vi "get_variable.vi"(4 "deviceName":string, 6 "timeout (ms)":i32=10000, 7 "IP address":string, 8 "error in (no error)":errorcluster, 9 "token cluster in":T1, 10 "variable name":string, 11 "client handle":T2) -> (0 "error out":errorcluster, 1 "token cluster":T1, 2 "variable value":string, 3 "client handle out":T2)   [LabVIEW 2018]
uses:
  <vilib>/httpClient/ClientHandle.ctl
  <vilib>/httpClient/LabVIEWHTTPClient.lvlib
panel:
  out "url":string
  out "headers":string
  out "status code":string
  out "msg":string
  out "reponse":string
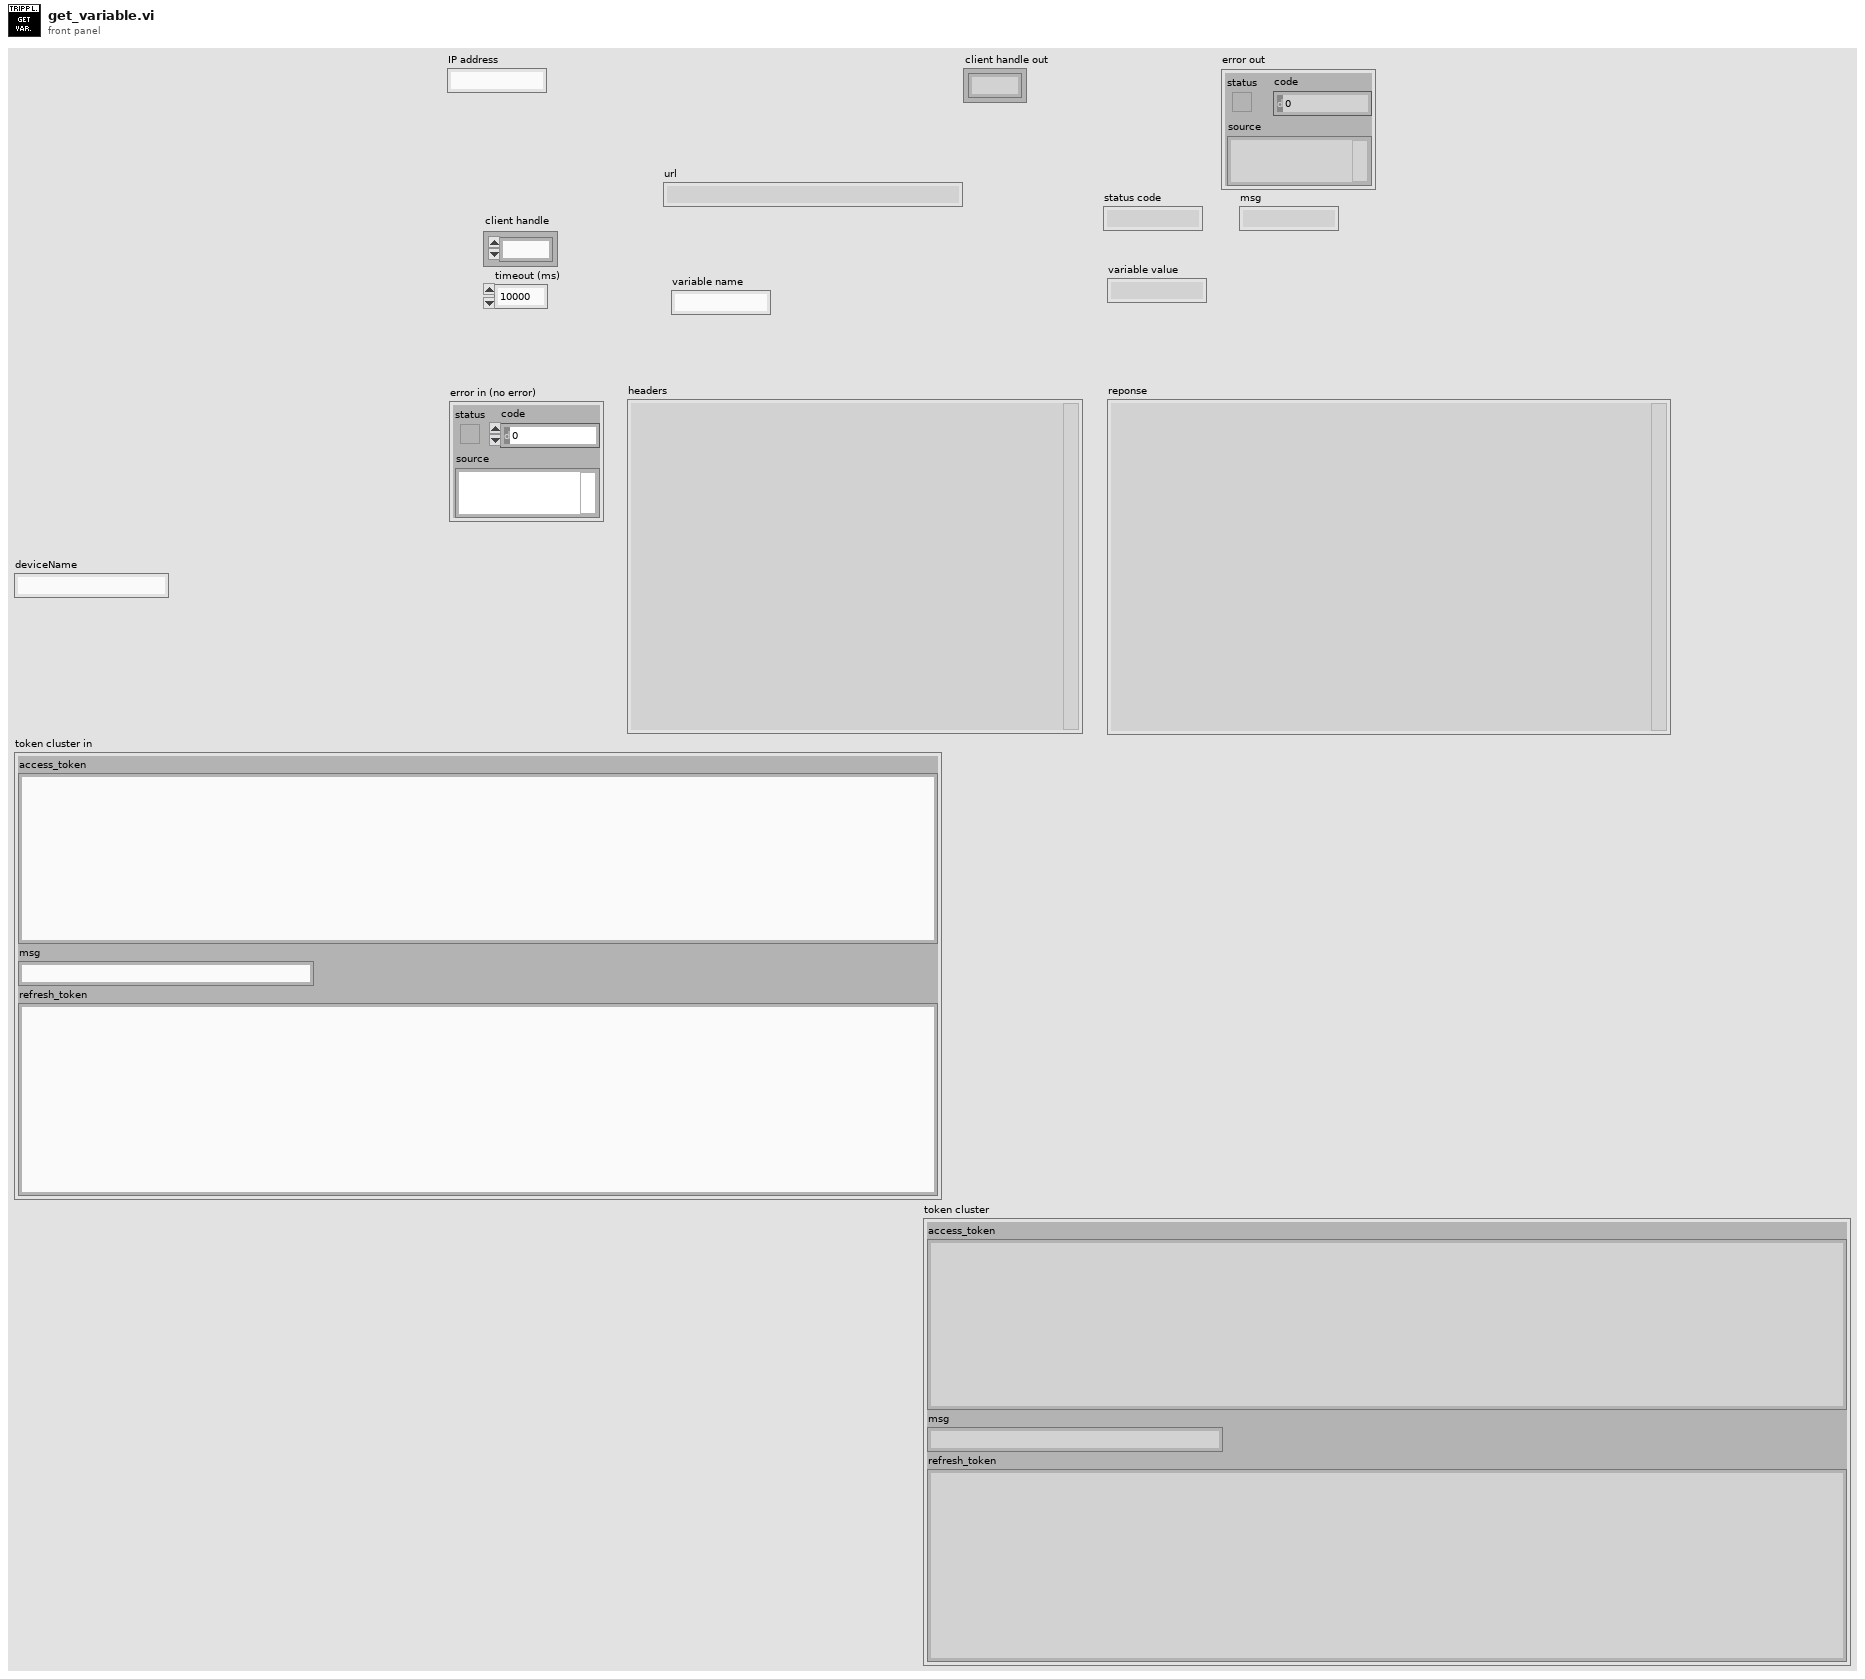
[diagram p1: front panel]
types:
  T1 = cluster{"access_token":string, "msg":string, "refresh_token":string}
  T2 = typedef "LabVIEWHTTPClient.lvlib/ClientHandle.ctl" = refnum<k1>
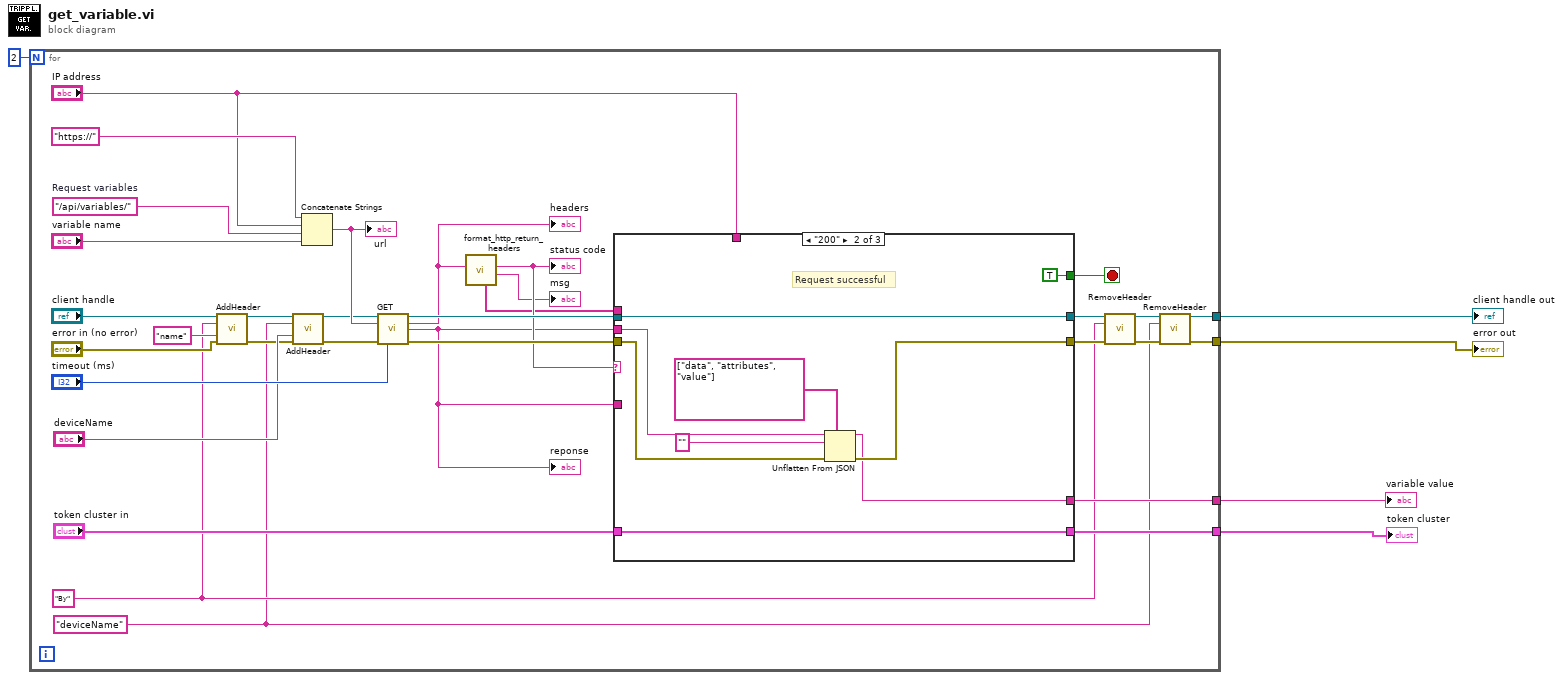
[diagram p0: block diagram]
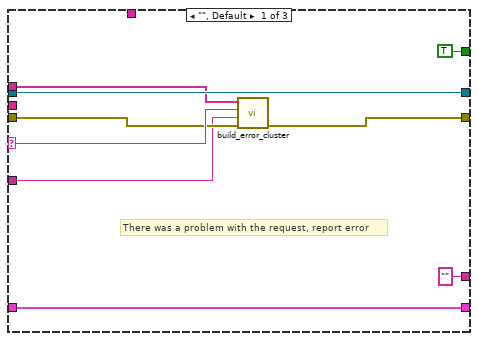
[diagram p2: hidden frame]
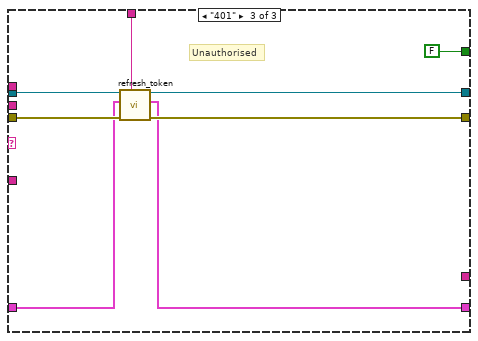
[diagram p3: hidden frame]
diagram:
  n1 = for {
    N: 2 -> [_]
    tunnel: [w6] -> w5
    tunnel: [w7] -> w4
    tunnel: [w28] -> w3
    tunnel: [w24] -> w1
    stop <- w22 stop-if-true
    w8 = "deviceName"
    w9 = "By"
    w35 = "/api/variables/"  # Request variables
    n2 = call <vilib>:"AddHeader.vi"("client handle"="client handle", "header"=w9, "value"="name", "error in (no error)"="error in (no error)") -> ("client handle out"=w13:T2, "error out"=w12:errorcluster)  [unwired: 10 in]
    n3 = call <vilib>:"AddHeader.vi"("client handle"=w13, "header"=w8, "value"="deviceName", "error in (no error)"=w12) -> ("client handle out"=w10:T2, "error out"=w11:errorcluster)  [unwired: 10 in]
    n4 = Concatenate Strings("https://", "IP address", w35, "variable name") -> (w38:string)
    "url" <- w38
    n5 = call <vilib>:"GET.vi"("client handle"=w10, "url"=w38, "error in (no error)"=w11, "timeout (10000)"="timeout (ms)") -> ("client handle out"=w36:T2, "headers"=w33:string, "body"=w27:string, "error out"=w37:errorcluster)  [unwired: 8 in]
    "reponse" <- w27
    "headers" <- w33
    n6 = call "format_http_return_headers.vi"("headers in"=w33) -> ("msg"=→"msg":string, "status code"=w32:string, "headers array"=w30:string[])  [unwired: 8 in]
    "status code" <- w32
    n7 = case shown="\"200\"" w32 {
      selector: w32 -> [w46 _ _]
      tunnel: w37 -> [w44 w51 w64]
      tunnel: w27 -> [_ w52 _]
      tunnel: w36 -> [w47 w56 w61]
      tunnel: [w43 w50 w63] -> w19
      tunnel: [w47 w56 w62] -> w20
      tunnel: ["" ("body") w49 _] -> w28
      tunnel: w30 -> [w45 _ _]
      tunnel: w27 -> [w41 _ _]
      tunnel: "token cluster in" -> [w39 w54 w60]
      tunnel: [w39 w54 w59] -> w24
      tunnel: "IP address" -> [_ _ w58]
      tunnel: [TRUE TRUE FALSE] -> w22
      frame "", Default {
        # "There was a problem with the request, report error"
        n8 = call "build_error_cluster.vi"("error in (no error)"=w44, "error msg (JSON)"=w41, "status code"=w46, "headers array"=w45) -> ("error out"=w43:errorcluster)  [unwired: 7 in]
      }
      frame "200" {
        # "Request successful"
        n9 = Unflatten From JSON(path=string[] ["data", "attributes", "value"], JSON string=w52, type and defaults="", error in (no error)=w51) -> (value=w49:string, error out=w50:errorcluster)  [unwired: 3 in]
      }
      frame "401" {
        # "Unauthorised"
        n10 = call "refresh_token.vi"("IP address"=w58, "error in (no error)"=w64, "token cluster in"=w60, "client handle"=w61) -> ("error out"=w63:errorcluster, "token cluster"=w59:T1, "client handle out"=w62:T2)  [unwired: 5 in]
      }
    }
    n11 = call <vilib>:"RemoveHeader.vi"("client handle"=w20, "header"=w9, "error in (no error)"=w19) -> ("client handle out"=w18:T2, "error out"=w17:errorcluster)  [unwired: 11 in]
    n12 = call <vilib>:"RemoveHeader.vi"("client handle"=w18, "header"=w8, "error in (no error)"=w17) -> ("client handle out"=w7:T2, "error out"=w6:errorcluster)  [unwired: 11 in]
  }
  "error out" <- w5
  "client handle out" <- w4
  "variable value" <- w3
  "token cluster" <- w1
